vi "ShowErrorDETVI.vi"(8 "error in (no error)":errorcluster, 11 "Detector in":refnum<class "Detector.lvclass">) -> (0 "error out":errorcluster, 3 "Detector out":refnum<class "Detector.lvclass">)   [LabVIEW 2020, in "Detector.lvclass"]
uses:
  Detector.lvclass
  C:/dev/TRANCON/Classes/GeneralFunctionality/GeneralFunctionality.lvclass
  GeneralFunctionality/GeneralFunctionality.lvclass/GeneralFunctionality.ctl
  GeneralFunctionality/GeneralFunctionality.lvclass
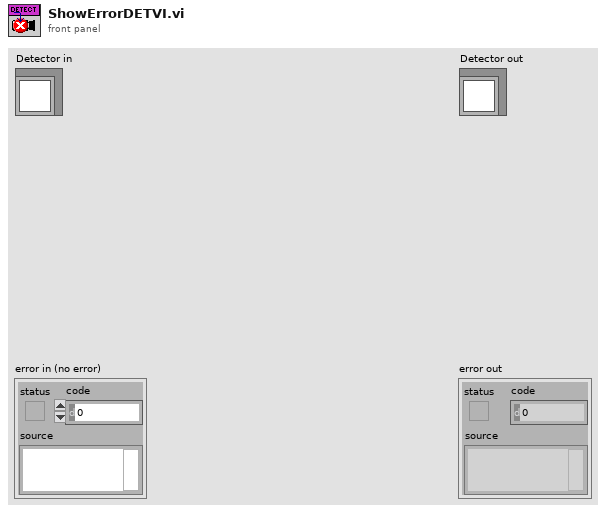
[diagram p1: front panel]
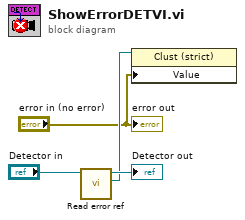
[diagram p0: block diagram]
diagram:
  n1 = call "Read error ref.vi"("GeneralFunctionality in"="Detector in") -> ("error"=w2:refnum<vi>, "GeneralFunctionality out"=→"Detector out":refnum<class "Detector.lvclass">)  [unwired: 8 in, 1 out]
  n2 = property class="Clust (strict)"(reference=w2, "Value"="error in (no error)") -> ()  [unwired: 1 in, 2 out]
  "error out" <- "error in (no error)"
